vi "Create Named FIFOs.vi"(8 "error in (no error)":errorcluster, 10 "DataRef Array":T3(array[cluster]) {"Block Data Refs"."Data Reference" format="%.0x"}, 11 "FIFO Name":string) -> (0 "error out":errorcluster, 2 "FIFO Names":string[](array[string]), 3 "FIFOs":refnum<k33>[](array[refnum]))   [LabVIEW 2017, in "Shared Variables CD 2.0 Engine.lvlib"]
uses:
  Shared Variables CD 2.0 Engine.lvlib
  <vilib>/NI Veristand/Custom Device API/Data Reference.ctl
  <vilib>/NI Veristand/Custom Device API/Custom Device API.lvlib
  <vilib>/NI Veristand/Custom Device API/Block Data Reference.ctl
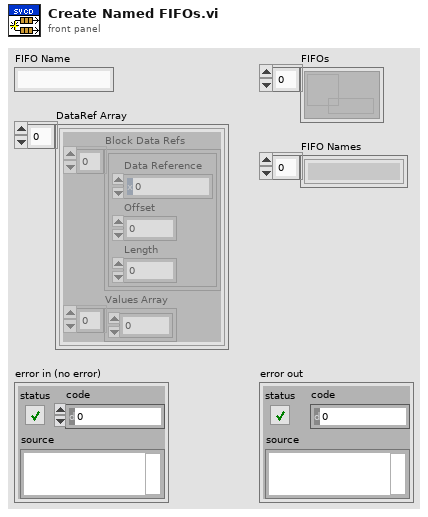
[diagram p1: front panel]
types:
  T1 = typedef "Custom Device API.lvlib/Block Data Reference.ctl" = cluster{"Data Reference":T2, "Offset":u64, "Length":u64}
  T2 = typedef "Custom Device API.lvlib/Data Reference.ctl" = i32
  T3 = cluster{"Block Data Refs":T1[], "Values Array":dbl[]}[]
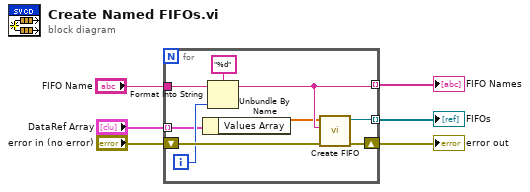
[diagram p0: block diagram]
diagram:
  n1 = for {
    tunnel: [w13] -> w4 mode=indexing
    shift-right: [w14] -> w5
    shift-left: "error in (no error)" -> [w15]
    tunnel: "DataRef Array" -> [w8] mode=indexing
    tunnel: "FIFO Name" -> [w12]
    tunnel: [w10] -> w6 mode=indexing
    i -> [w11]
    n2 = Unbundle By Name(w8) -> ("Values Array"=w7:dbl[])
    n3 = Format Into String(format string="%d", initial string=w12, w11) -> (resulting string=w10:string)  [unwired: 1 in, 1 out]
    n4 = call "Create FIFO.vi"("error in (no error)"=w15, "DataRef"=w10, "FIFO Name"=w7) -> ("error out"=w14:errorcluster, "FIFO Ref"=w13:refnum<k33>)  [unwired: 7 in]
  }
  "FIFO Names" <- w6
  "error out" <- w5
  "FIFOs" <- w4
